vi "Settings_Hardware_FGV.vi"(7 "Command":T5(ring), 8 "error in (no error)":errorcluster, 10 "XML Path":path=path "D:/TEST.xml", 11 "Variant":variant) -> (0 "error out":errorcluster, 1 "HARDWARE Inputs in String":T4 {"AO 6711 Inputs"."Max Voltage" min=-10.0 max=10.0; "AO 6711 Inputs"."Min Voltage" min=-10.0 max=10.0}, 2 "XML String Out":string[](array[string]), 3 "Variant Output":variant)   [LabVIEW 2015]
doc: "This VI reads an XML file of parameters and casts the Resource Name (String) to an IVI Class, as the GXML Lib is unable to read/write objects of type IVI class."
uses:
  controls/AO_6711_Inputs.ctl
  <instrlib>/niHSDIO/niHSDIO.llb/niHSDIO_ctl Trigger Source Values (Ring).ctl
  <instrlib>/niScope/Controls/niScope trigger source.ctl
  controls/HARDWARE_Inputs.ctl
  controls/AWG_5421_Inputs.ctl
  controls/DIGIT_5122_Inputs.ctl
  controls/HSDIO_6541_Inputs.ctl
  <vilib>/NI/GXML/_subVIs/GXML SearchParser/Search Parser.vi
  <vilib>/NI/GXML/GXML.lvlib
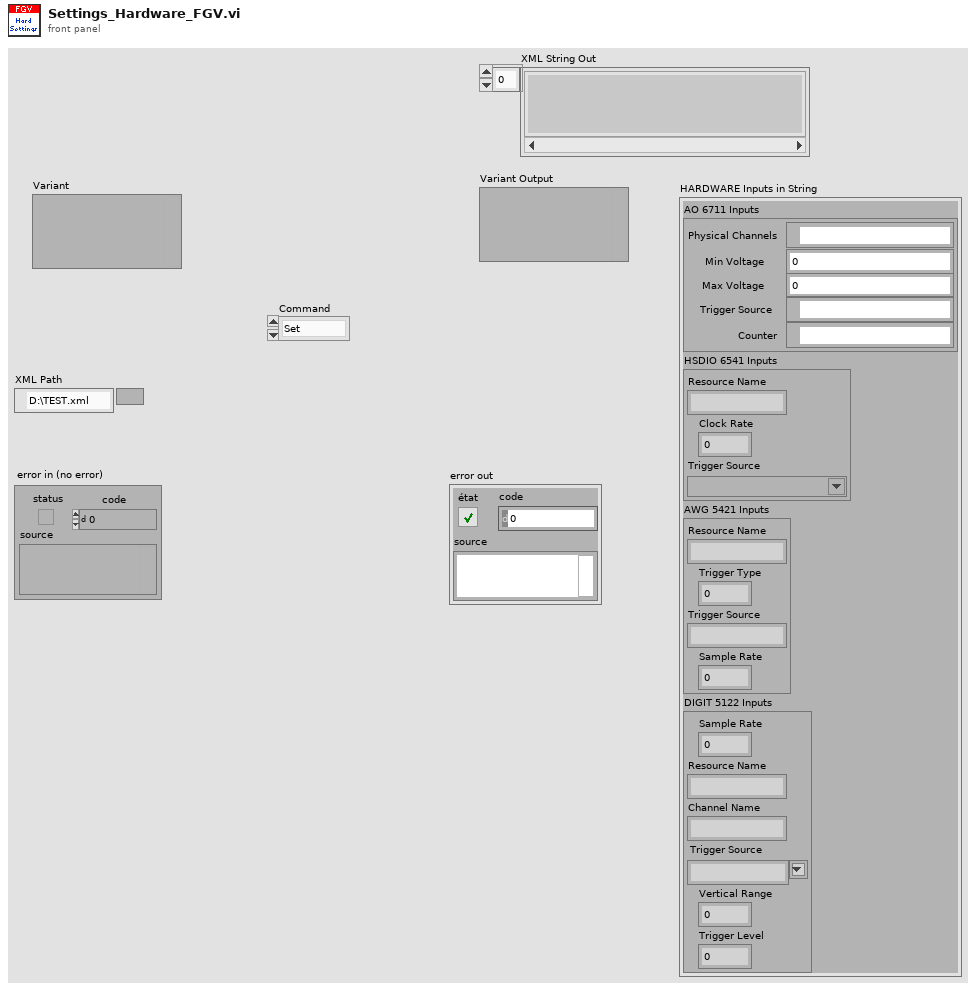
[diagram p1: front panel]
types:
  T1 = typedef "AO_6711_Inputs.ctl" = cluster{"Physical Channels":tag, "Min Voltage":dbl, "Max Voltage":dbl, "Trigger Source":tag, "counter":tag}
  T2 = typedef "niHSDIO_ctl Trigger Source Values (Ring).ctl" = string
  T3 = typedef "niScope trigger source.ctl" = string
  T4 = cluster{"AO 6711 Inputs":T1, "HSDIO 6541 Inputs":cluster{"Resource Name":string, "Clock Rate":dbl, "Trigger Source":T2}, "AWG 5421 Inputs":cluster{"Resource Name":string, "Trigger Type":u16, "Trigger Source":string, "Sample Rate":dbl}, "DIGIT 5122 Inputs":cluster{"Sample Rate":dbl, "Resource Name":string, "Channel Name":string, "Trigger Source":T3, "Vertical Range":dbl, "Trigger Level":dbl}}
  T5 = enum16{"Set", "Get", "Read XML", "Write XML", "Convert to String"}
  T6 = typedef "HARDWARE_Inputs.ctl" = cluster{"AO 6711 Inputs":T1, "AWG 5421 Inputs":T7, "DIGIT 5122 Inputs":T8, "HSDIO 6541 Inputs":T9}
  T7 = typedef "AWG_5421_Inputs.ctl" = cluster{"Resource Name":refnum<k15>, "Trigger Type":u16, "Trigger Source":string, "Sample Rate":dbl}
  T8 = typedef "DIGIT_5122_Inputs.ctl" = cluster{"Sample Rate":dbl, "Resource Name":refnum<k15>, "Channel Name":string, "Trigger Source":T3, "Vertical Range":dbl, "Trigger Level":dbl}
  T9 = typedef "HSDIO_6541_Inputs.ctl" = cluster{"Resource Name":refnum<k15>, "Clock Rate":dbl, "Trigger Source":T2}
  T10 = cluster{"Sample Rate":dbl, "Resource Name":string, "Channel Name":string, "Trigger Source":T3, "Vertical Range":dbl, "Trigger Level":dbl}
  T11 = cluster{"Resource Name":string, "Trigger Type":u16, "Trigger Source":string, "Sample Rate":dbl}
  T12 = cluster{"Resource Name":string, "Clock Rate":dbl, "Trigger Source":T2}
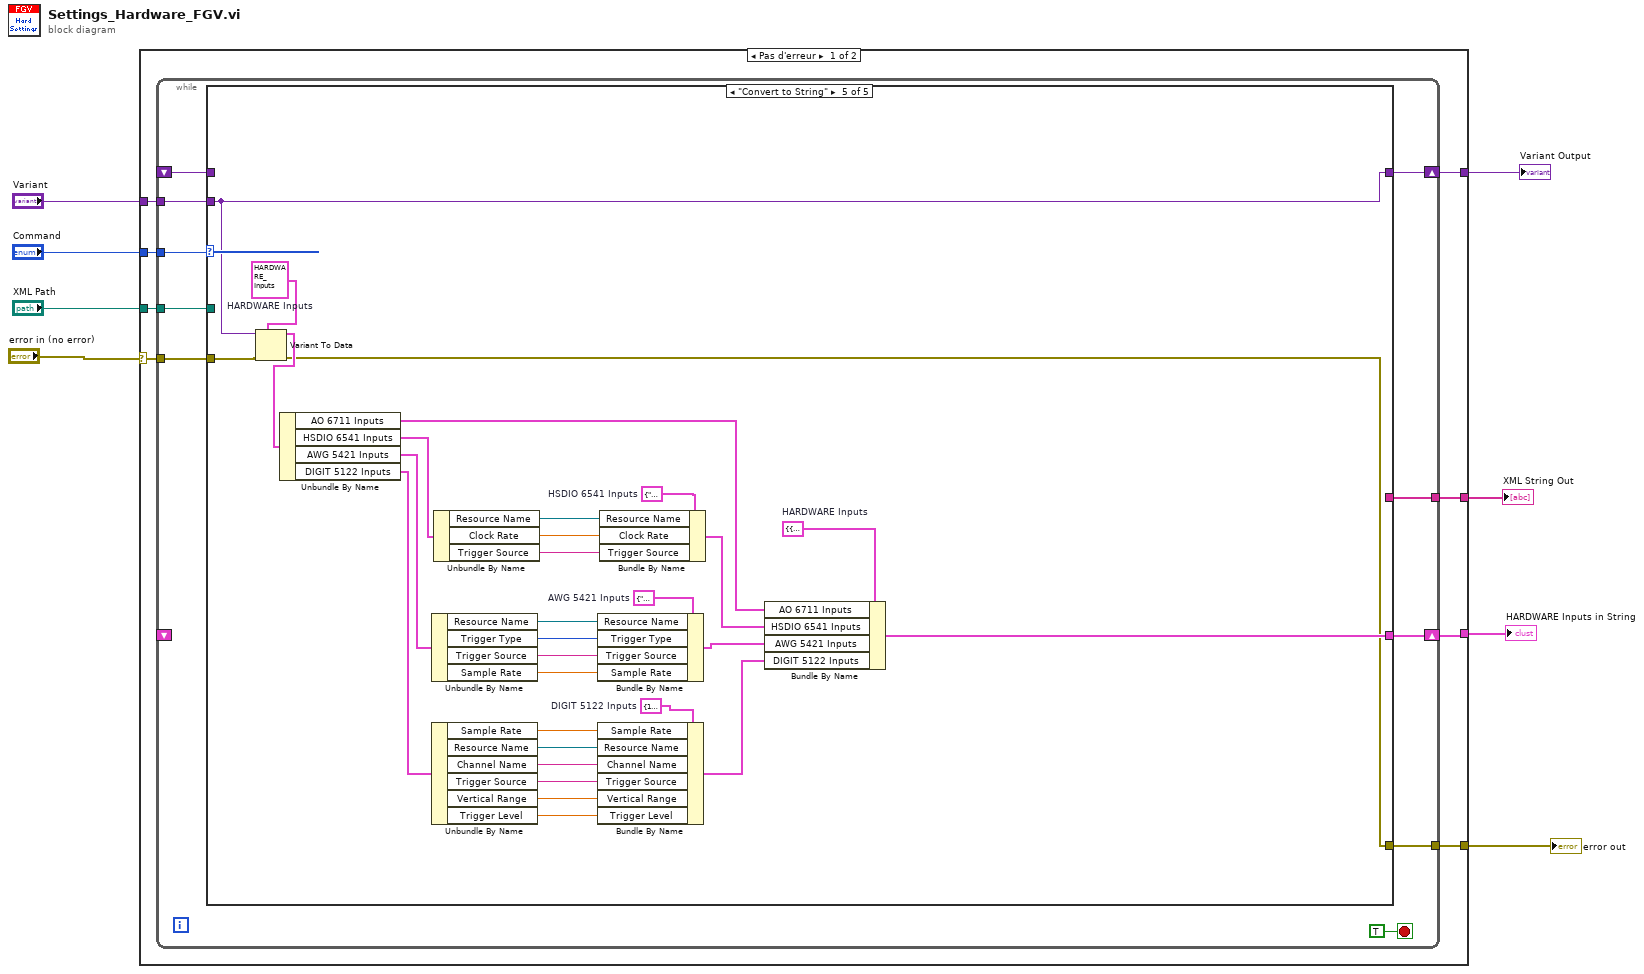
[diagram p0: block diagram]
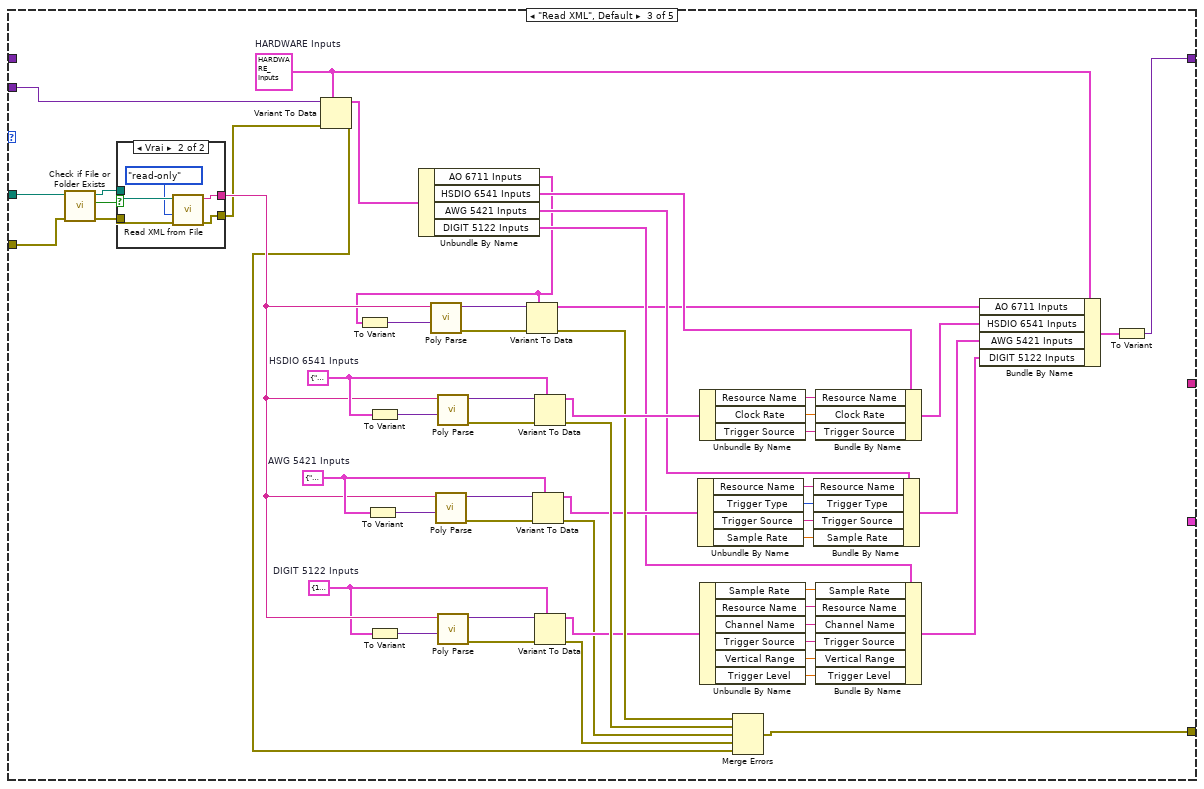
[diagram p4: hidden frame]
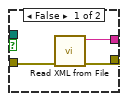
[diagram p5: hidden frame]
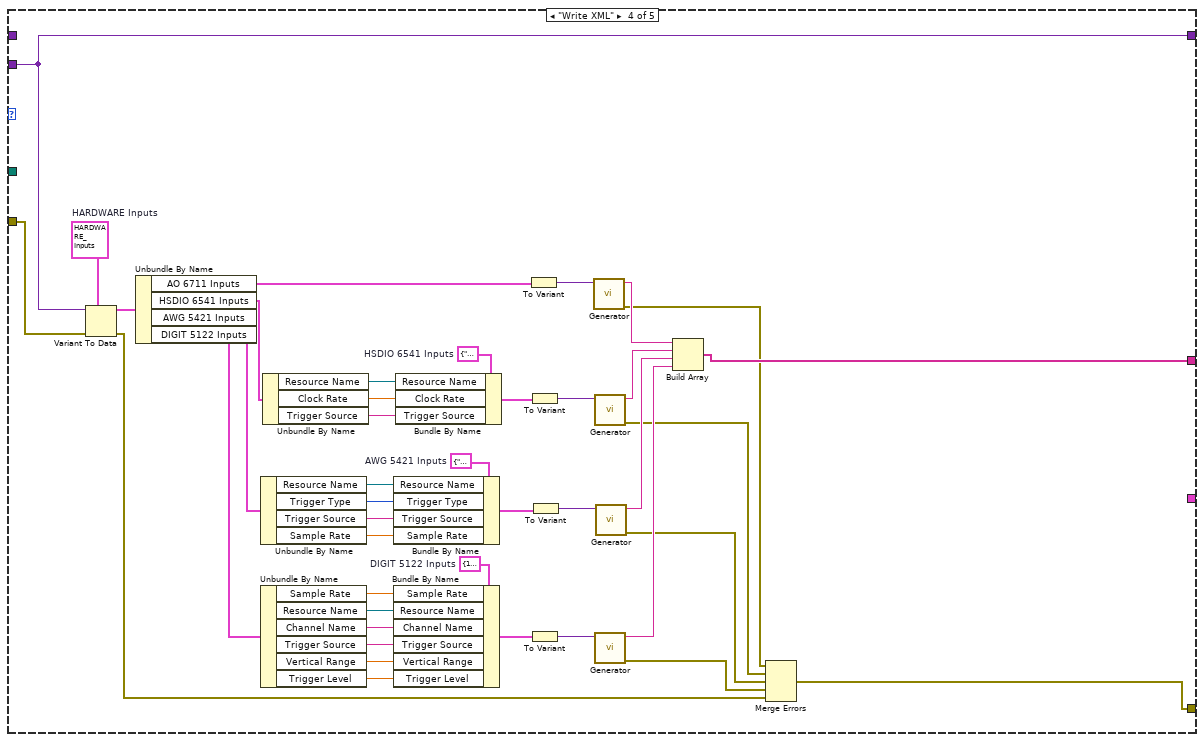
[diagram p6: hidden frame]
diagram:
  n1 = case shown="Pas d'erreur" "error in (no error)" {
    selector: "error in (no error)" -> [w15 w169]
    tunnel: "Command" -> [w16 _]
    tunnel: [w14 w169] -> w6
    tunnel: "XML Path" -> [w13 _]
    tunnel: [w12 w168] -> w3
    tunnel: [w11 _] -> w4
    tunnel: "Variant" -> [w10 w168]
    tunnel: [w9 _] -> w1
    frame No Error {
      n2 = while {
        tunnel: w16 -> [w25]
        tunnel: w15 -> [w24]
        tunnel: [w23] -> w14
        tunnel: w13 -> [w22]
        shift-right: [w19] -> w12
        shift-left: _ -> [w18]
        shift-right: [w21] -> w11
        shift-left: _ -> [_]
        tunnel: w10 -> [w20]
        tunnel: [w17] -> w9
        stop <- TRUE stop-if-true
        n3 = case shown="\"Convert to String\"" w25 {
          tunnel: w24 -> [w28 w30 w84 w116 w141]
          tunnel: [w28 w30 w69 w96 w140] -> w23
          tunnel: w22 -> [_ _ w81 _ _]
          tunnel: [_ _ _ _ w143] -> w21
          tunnel: w20 -> [w27 _ w37 w115 w138]
          tunnel: [w27 w29 w32 w115 w138] -> w19
          tunnel: w18 -> [_ w29 _ _ _]
          tunnel: [_ _ _ w102 _] -> w17
          frame "Set" {
          }
          frame "Get" {
          }
          frame "Read XML", Default {
            w33 = T6 {"AO 6711 Inputs"={"Physical Channels"="AnalogOutput/ao0:3", "Min Voltage"=-10.0, "Max Voltage"=10.0, "Trigger Source"="/AnalogOutput/PFI0", "counter"="AnalogOutput/ctr0"}, "AWG 5421 Inputs"={"Resource Name"="AnalogOutput/ao0:3", "Trigger Type"=2, "Trigger Source"="PFI0", "Sample Rate"=20000000.0}, "DIGIT 5122 Inputs"={"Sample Rate"=10000000.0, "Resource Name"="Digitizer", "Channel Name"="PFI0", "Trigger Source"="VAL_EXTERNAL", "Vertical Range"=10.0, "Trigger Level"=3.0}, "HSDIO 6541 Inputs"={"Resource Name"="SequencerHSDIO", "Clock Rate"=1000000.0, "Trigger Source"="PFI0"}}  # HARDWARE Inputs
            w46 = T10 {"Sample Rate"=10000000.0, "Resource Name"="Digitizer", "Channel Name"="0", "Trigger Source"="VAL_EXTERNAL", "Vertical Range"=10.0, "Trigger Level"=3.0}  # DIGIT 5122 Inputs
            w61 = T11 {"Resource Name"="WaveformGenerator", "Trigger Type"=2, "Trigger Source"="PFI0", "Sample Rate"=20000000.0}  # AWG 5421 Inputs
            w72 = T12 {"Resource Name"="SequencerHSDIO", "Clock Rate"=1000000.0, "Trigger Source"="PFI0"}  # HSDIO 6541 Inputs
            n4 = call <vilib>:"Check if File or Folder Exists.vi"("error in (no error)"=w84, "path"=w81) -> ("error out"=w87:errorcluster, "file or folder exists?"=w86:bool, "dup path"=w85:path)  [unwired: 7 in]
            n5 = case shown="Vrai" w86 {
              tunnel: w85 -> [_ w95]
              tunnel: w87 -> [w90 w93]
              tunnel: [w88 w94] -> w54
              tunnel: [w89 w92] -> w35
              frame False {
                n6 = call <vilib>:"Read XML from File.vi"("error in"=w90) -> ("error out"=w89:errorcluster, "XML String Out"=w88:string)  [unwired: 9 in]
              }
              frame True {
                n7 = call <vilib>:"Read XML from File.vi"("error in"=w93, "file access"=enum16{"read/write", "read-only", "write-only"}."read-only", "XML File Path"=w95) -> ("error out"=w92:errorcluster, "XML String Out"=w94:string)  [unwired: 7 in]
              }
            }
            n8 = Variant To Data(error in=w35, type=w33, Variant=w37) -> (data=w36:T6, error out=w34:errorcluster)
            n9 = To Variant(anything=w61) -> (Variant=w68:variant)
            n10 = To Variant(anything=w72) -> (Variant=w80:variant)
            n11 = To Variant(anything=w46) -> (Variant=w60:variant)
            n12 = Unbundle By Name(w36) -> ("AO 6711 Inputs"=w42:T1, "HSDIO 6541 Inputs"=w45:T9, "AWG 5421 Inputs"=w44:T7, "DIGIT 5122 Inputs"=w43:T8)
            n13 = To Variant(anything=w42) -> (Variant=w77:variant)
            n14 = call-poly <vilib>:"Poly Parse.vi"("TypeDesc"=w77, "XML String In"=w54) -> ("error out"=w82:errorcluster, "Parsed Data"=w83:variant)  [unwired: 8 in]
            n15 = call-poly <vilib>:"Poly Parse.vi"("TypeDesc"=w68, "XML String In"=w54) -> ("error out"=w67:errorcluster, "Parsed Data"=w66:variant)  [unwired: 8 in]
            n16 = call-poly <vilib>:"Poly Parse.vi"("TypeDesc"=w80, "XML String In"=w54) -> ("error out"=w79:errorcluster, "Parsed Data"=w78:variant)  [unwired: 8 in]
            n17 = call-poly <vilib>:"Poly Parse.vi"("TypeDesc"=w60, "XML String In"=w54) -> ("error out"=w59:errorcluster, "Parsed Data"=w58:variant)  [unwired: 8 in]
            n18 = Variant To Data(error in=w82, type=w42, Variant=w83) -> (data=w41:T1, error out=w71:errorcluster)
            n19 = Variant To Data(error in=w67, type=w61, Variant=w66) -> (data=w62:T11, error out=w48:errorcluster)
            n20 = Variant To Data(error in=w79, type=w72, Variant=w78) -> (data=w73:T12, error out=w70:errorcluster)
            n21 = Variant To Data(error in=w59, type=w46, Variant=w58) -> (data=w55:T10, error out=w47:errorcluster)
            n22 = Unbundle By Name(w62) -> ("Resource Name"=w63:string, "Trigger Type"=w65:u16, "Trigger Source"=w64:string, "Sample Rate"=w49:dbl)
            n23 = Unbundle By Name(w73) -> ("Resource Name"=w74:string, "Clock Rate"=w76:dbl, "Trigger Source"=w75:T2)
            n24 = Unbundle By Name(w55) -> ("Sample Rate"=w56:dbl, "Resource Name"=w53:string, "Channel Name"=w57:string, "Trigger Source"=w52:T3, "Vertical Range"=w51:dbl, "Trigger Level"=w50:dbl)
            n25 = Merge Errors(w71, w70, w48, w47, w34) -> (w69:errorcluster)
            n26 = Bundle By Name(cluster=w44, "Resource Name"=w63, "Trigger Type"=w65, "Trigger Source"=w64, "Sample Rate"=w49) -> (w38:T7)
            n27 = Bundle By Name(cluster=w45, "Resource Name"=w74, "Clock Rate"=w76, "Trigger Source"=w75) -> (w40:T9)
            n28 = Bundle By Name(cluster=w43, "Sample Rate"=w56, "Resource Name"=w53, "Channel Name"=w57, "Trigger Source"=w52, "Vertical Range"=w51, "Trigger Level"=w50) -> (w39:T8)
            n29 = Bundle By Name(cluster=w33, "AO 6711 Inputs"=w41, "HSDIO 6541 Inputs"=w40, "AWG 5421 Inputs"=w38, "DIGIT 5122 Inputs"=w39) -> (w31:T6)
            n30 = To Variant(anything=w31) -> (Variant=w32:variant)
          }
          frame "Write XML" {
            w118 = T6 {"AO 6711 Inputs"={"Physical Channels"="AnalogOutput/ao0:3", "Min Voltage"=-10.0, "Max Voltage"=10.0, "Trigger Source"="/AnalogOutput/PFI0", "counter"="AnalogOutput/ctr0"}, "AWG 5421 Inputs"={"Resource Name"="AnalogOutput/ao0:3", "Trigger Type"=2, "Trigger Source"="PFI0", "Sample Rate"=20000000.0}, "DIGIT 5122 Inputs"={"Sample Rate"=10000000.0, "Resource Name"="Digitizer", "Channel Name"="PFI0", "Trigger Source"="VAL_EXTERNAL", "Vertical Range"=10.0, "Trigger Level"=3.0}, "HSDIO 6541 Inputs"={"Resource Name"="SequencerHSDIO", "Clock Rate"=1000000.0, "Trigger Source"="PFI0"}}  # HARDWARE Inputs
            w135 = T10 {"Sample Rate"=10000000.0, "Resource Name"="Digitizer", "Channel Name"="0", "Trigger Source"="VAL_EXTERNAL", "Vertical Range"=10.0, "Trigger Level"=3.0}  # DIGIT 5122 Inputs
            w136 = T11 {"Resource Name"="WaveformGenerator", "Trigger Type"=2, "Trigger Source"="PFI0", "Sample Rate"=20000000.0}  # AWG 5421 Inputs
            w137 = T12 {"Resource Name"="SequencerHSDIO", "Clock Rate"=1000000.0, "Trigger Source"="PFI0"}  # HSDIO 6541 Inputs
            n31 = Variant To Data(error in=w116, type=w118, Variant=w115) -> (data=w117:T6, error out=w97:errorcluster)
            n32 = Unbundle By Name(w117) -> ("AO 6711 Inputs"=w113:T1, "HSDIO 6541 Inputs"=w132:T9, "AWG 5421 Inputs"=w133:T7, "DIGIT 5122 Inputs"=w134:T8)
            n33 = Unbundle By Name(w133) -> ("Resource Name"=w125:refnum<k15>, "Trigger Type"=w124:u16, "Trigger Source"=w123:string, "Sample Rate"=w122:dbl)
            n34 = Unbundle By Name(w134) -> ("Sample Rate"=w131:dbl, "Resource Name"=w130:refnum<k15>, "Channel Name"=w129:string, "Trigger Source"=w128:T3, "Vertical Range"=w127:dbl, "Trigger Level"=w126:dbl)
            n35 = Unbundle By Name(w132) -> ("Resource Name"=w119:refnum<k15>, "Clock Rate"=w120:dbl, "Trigger Source"=w121:T2)
            n36 = Bundle By Name(cluster=w136, "Resource Name"=w125, "Trigger Type"=w124, "Trigger Source"=w123, "Sample Rate"=w122) -> (w107:T11)
            n37 = Bundle By Name(cluster=w135, "Sample Rate"=w131, "Resource Name"=w130, "Channel Name"=w129, "Trigger Source"=w128, "Vertical Range"=w127, "Trigger Level"=w126) -> (w105:T10)
            n38 = Bundle By Name(cluster=w137, "Resource Name"=w119, "Clock Rate"=w120, "Trigger Source"=w121) -> (w110:T12)
            n39 = To Variant(anything=w113) -> (Variant=w114:variant)
            n40 = To Variant(anything=w110) -> (Variant=w111:variant)
            n41 = To Variant(anything=w105) -> (Variant=w106:variant)
            n42 = To Variant(anything=w107) -> (Variant=w108:variant)
            n43 = call <vilib>:"Generator.vi"("Variant"=w114) -> ("error out"=w101:errorcluster, "XML String Out"=w112:string)  [unwired: 9 in]
            n44 = call <vilib>:"Generator.vi"("Variant"=w111) -> ("error out"=w100:errorcluster, "XML String Out"=w109:string)  [unwired: 9 in]
            n45 = call <vilib>:"Generator.vi"("Variant"=w106) -> ("error out"=w98:errorcluster, "XML String Out"=w103:string)  [unwired: 9 in]
            n46 = call <vilib>:"Generator.vi"("Variant"=w108) -> ("error out"=w99:errorcluster, "XML String Out"=w104:string)  [unwired: 9 in]
            n47 = Build Array(w112, w109, w104, w103) -> (w102:string[])
            n48 = Merge Errors(w101, w100, w99, w98, w97) -> (w96:errorcluster)
          }
          frame "Convert to String" {
            w139 = T6 {"AO 6711 Inputs"={"Physical Channels"="AnalogOutput/ao0:3", "Min Voltage"=-10.0, "Max Voltage"=10.0, "Trigger Source"="/AnalogOutput/PFI0", "counter"="AnalogOutput/ctr0"}, "AWG 5421 Inputs"={"Resource Name"="WaveformGenerator", "Trigger Type"=2, "Trigger Source"="PFI0", "Sample Rate"=20000000.0}, "DIGIT 5122 Inputs"={"Sample Rate"=10000000.0, "Resource Name"="Digitizer", "Channel Name"="0", "Trigger Source"="VAL_EXTERNAL", "Vertical Range"=10.0, "Trigger Level"=3.0}, "HSDIO 6541 Inputs"={"Resource Name"="SequencerHSDIO", "Clock Rate"=1000000.0, "Trigger Source"="PFI0"}}  # HARDWARE Inputs
            w142 = T4 {"AO 6711 Inputs"={"Physical Channels"="AnalogOutput/ao0:3", "Min Voltage"=-10.0, "Max Voltage"=10.0, "Trigger Source"="/AnalogOutput/PFI0", "counter"="AnalogOutput/ctr0"}, "HSDIO 6541 Inputs"={"Resource Name"="SequencerHSDIO", "Clock Rate"=1000000.0, "Trigger Source"="PFI0"}, "AWG 5421 Inputs"={"Resource Name"="WaveformGenerator", "Trigger Type"=2, "Trigger Source"="PFI0", "Sample Rate"=20000000.0}, "DIGIT 5122 Inputs"={"Sample Rate"=10000000.0, "Resource Name"="Digitizer", "Channel Name"="0", "Trigger Source"="VAL_EXTERNAL", "Vertical Range"=10.0, "Trigger Level"=3.0}}  # HARDWARE Inputs
            w165 = T10 {"Sample Rate"=10000000.0, "Resource Name"="Digitizer", "Channel Name"="0", "Trigger Source"="VAL_EXTERNAL", "Vertical Range"=10.0, "Trigger Level"=3.0}  # DIGIT 5122 Inputs
            w166 = T11 {"Resource Name"="WaveformGenerator", "Trigger Type"=2, "Trigger Source"="PFI0", "Sample Rate"=20000000.0}  # AWG 5421 Inputs
            w167 = T12 {"Resource Name"="SequencerHSDIO", "Clock Rate"=1000000.0, "Trigger Source"="PFI0"}  # HSDIO 6541 Inputs
            n49 = Variant To Data(error in=w141, type=w139, Variant=w138) -> (data=w144:T6, error out=w140:errorcluster)
            n50 = Unbundle By Name(w144) -> ("AO 6711 Inputs"=w145:T1, "HSDIO 6541 Inputs"=w159:T9, "AWG 5421 Inputs"=w160:T7, "DIGIT 5122 Inputs"=w161:T8)
            n51 = Unbundle By Name(w160) -> ("Resource Name"=w152:refnum<k15>, "Trigger Type"=w151:u16, "Trigger Source"=w150:string, "Sample Rate"=w149:dbl)
            n52 = Unbundle By Name(w161) -> ("Sample Rate"=w158:dbl, "Resource Name"=w157:refnum<k15>, "Channel Name"=w156:string, "Trigger Source"=w155:T3, "Vertical Range"=w154:dbl, "Trigger Level"=w153:dbl)
            n53 = Unbundle By Name(w159) -> ("Resource Name"=w146:refnum<k15>, "Clock Rate"=w147:dbl, "Trigger Source"=w148:T2)
            n54 = Bundle By Name(cluster=w166, "Resource Name"=w152, "Trigger Type"=w151, "Trigger Source"=w150, "Sample Rate"=w149) -> (w163:T11)
            n55 = Bundle By Name(cluster=w165, "Sample Rate"=w158, "Resource Name"=w157, "Channel Name"=w156, "Trigger Source"=w155, "Vertical Range"=w154, "Trigger Level"=w153) -> (w162:T10)
            n56 = Bundle By Name(cluster=w167, "Resource Name"=w146, "Clock Rate"=w147, "Trigger Source"=w148) -> (w164:T12)
            n57 = Bundle By Name(cluster=w142, "AO 6711 Inputs"=w145, "HSDIO 6541 Inputs"=w164, "AWG 5421 Inputs"=w163, "DIGIT 5122 Inputs"=w162) -> (w143:T4)
          }
        }
      }
    }
    frame Error {
    }
  }
  "error out" <- w6
  "HARDWARE Inputs in String" <- w4
  "Variant Output" <- w3
  "XML String Out" <- w1
